vi "Operation.vi"(0 "Multiplication in":refnum<class "Multiplication.lvclass">, 11 "Error In":errorcluster) -> (4 "Multiplication out":refnum<class "Multiplication.lvclass">, 15 "Error Out":errorcluster)   [LabVIEW 2020, in "Multiplication.lvclass"]
uses:
  Multiplication.lvclass
  Multiplication.lvclass/Multiplication.ctl
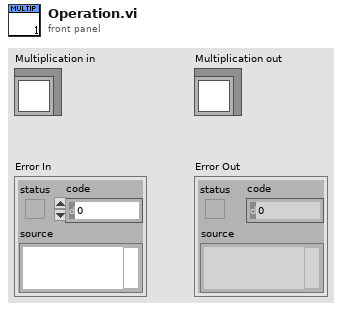
[diagram p1: front panel]
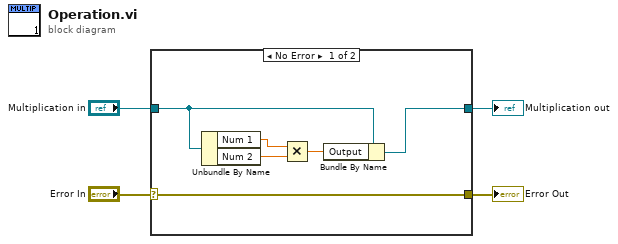
[diagram p0: block diagram]
diagram:
  n1 = case shown="No Error" "Error In" {
    selector: "Error In" -> [w10 w12]
    tunnel: [w10 w12] -> w3
    tunnel: [w6 w11] -> w1
    tunnel: "Multiplication in" -> [w9 w11]
    frame No Error {
      n2 = Unbundle By Name(w9) -> ("Num 1"=w7:dbl, "Num 2"=w8:dbl)
      n3 = Multiply(x=w7, y=w8) -> (x*y=w5:dbl)
      n4 = Bundle By Name(cluster=w9, "Output"=w5) -> (w6:refnum<class "Multiplication.lvclass">)
    }
    frame Error {
    }
  }
  "Error Out" <- w3
  "Multiplication out" <- w1
